vi "JYAddDevice.vi"(8 "error in (no error)":errorcluster) -> (0 "error out":errorcluster)   [LabVIEW 2009]
doc: "Invokes the JY Device Configuration Wizard. This allow devices to be registered and configured on the system. \n\nInputs - Input Error Cluster\nOutputs - Output Error Cluster"
panel:
  in  "JYDEVICECONFIGLib":refnum<k7>
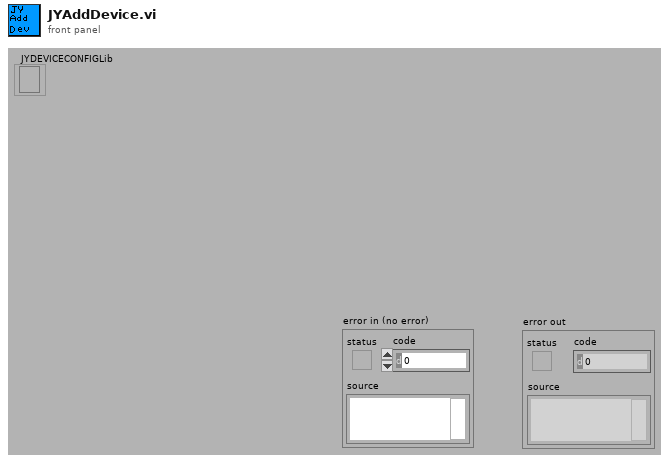
[diagram p1: front panel]
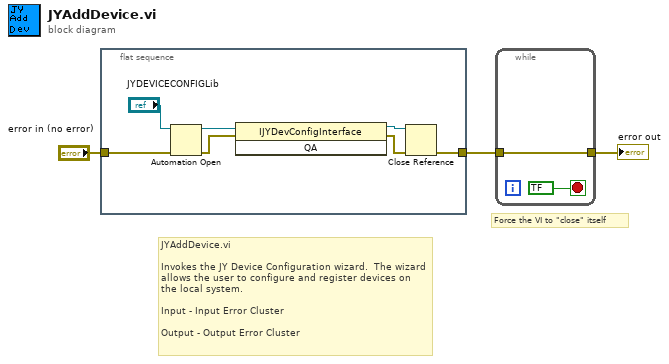
[diagram p0: block diagram]
diagram:
  # "JYAddDevice.vi\n\nInvokes the JY Device Configuration wizard.  The wizard\nallows the user to configure and register devices on \nthe local system.\n\nInput - Input Error Cluster\n\nOutput - Output Error Cluster"
  # "Force the VI to \"close\" itself"
  n1 = flat-sequence {
    tunnel: "error in (no error)" -> [w5]
    tunnel: [w4] -> w2
    frame #0 {
      n2 = Automation Open(error in (no error)=w5, Automation Refnum="JYDEVICECONFIGLib") -> (Automation Refnum=w9:refnum<k7>, error out=w7:errorcluster)  [unwired: 2 out]
      n3 = invoke class="IJYDevConfigInterface" method="QA"(reference=w9, error in=w7) -> (reference out=w8:refnum<k7>, error out=w6:errorcluster)  [unwired: 1 in, 1 out]
      n4 = Close Reference(reference=w8, error in (no error)=w6) -> (error out=w4:errorcluster)
    }
  }
  n5 = while {
    tunnel: w2 -> [w11]
    tunnel: [w11] -> w1
    stop <- bool ? stop-if-true
  }
  "error out" <- w1
